vi "pressSensorLin.vi"(0 "frame":u8[](array[numeric])) -> ()   [LabVIEW 2021]
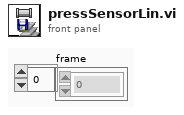
[diagram p1: front panel]
types:
  T1 = cluster{"ValvePos1":sgl, "ValvePos2":sgl, "PressureArray":sgl[], "TempArray2":sgl[], "TempArray1":sgl[], "Valve 1 Time Stamp":timestamp, "Temp 2 Array Time Stamp":timestamp[], "Temp 1 Array Time Stamp":timestamp[], "Valve 2 Time Stamp":timestamp, "Press Array Time Stamp":timestamp[]}
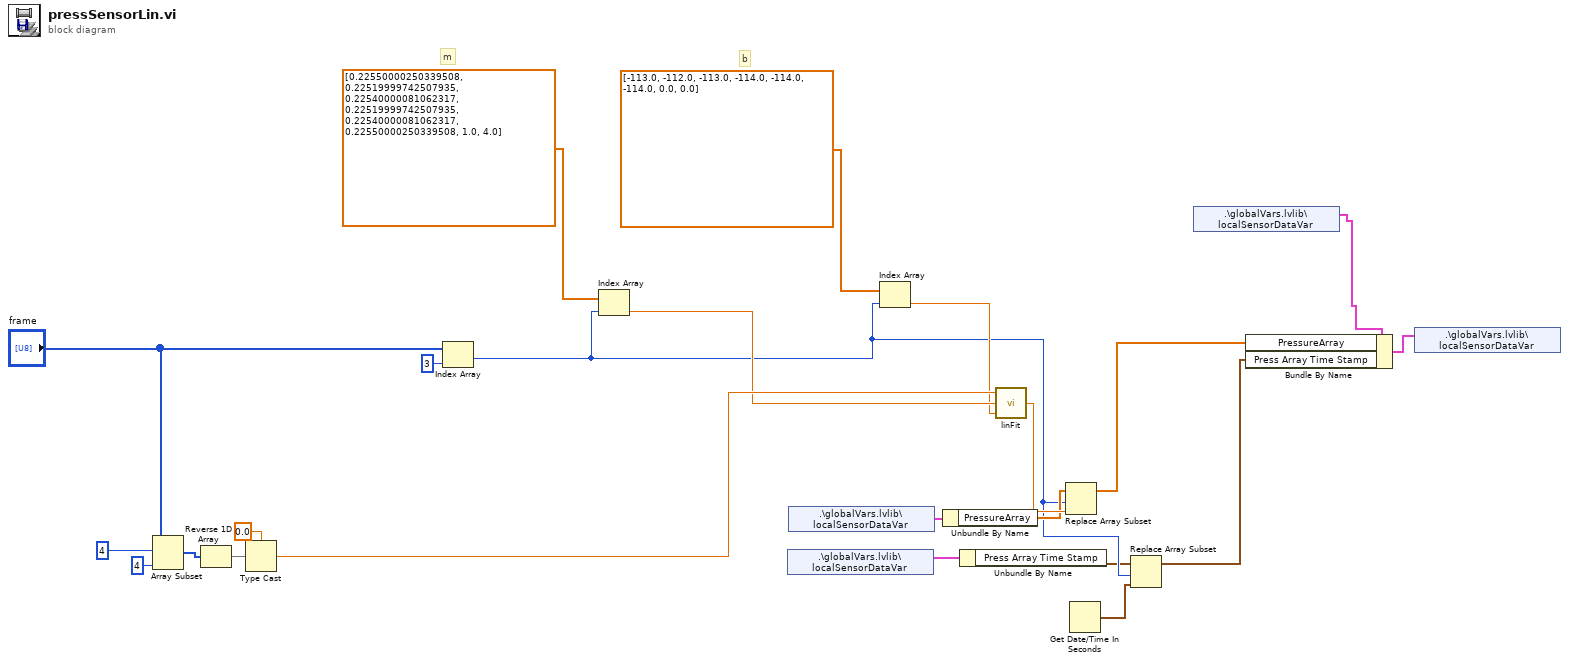
[diagram p0: block diagram]
diagram:
  # "b"
  # "m"
  n1 = Array Subset(array="frame", index=4, length=4) -> (w19:u8[])
  n2 = Reverse 1D Array(array=w19) -> (reversed array=w20:u8[])
  n3 = Type Cast(type=sgl 0.0, x=w20) -> (*(type *) &x=w14:sgl)
  n4 = Index Array(array="frame", index=3) -> (element=w5:u8)
  n5 = Index Array(array=sgl[] [0.2255, 0.2252, 0.2254, 0.2252, 0.2254, 0.2255, 1.0, 4.0], index=w5) -> (element=w13:sgl)
  n6 = shared-variable ".\\globalVars.lvlib\\localSensorDataVar"() -> (w6:T1)  [unwired: 1 in, 1 out]
  n7 = shared-variable ".\\globalVars.lvlib\\localSensorDataVar"() -> (w11:T1)  [unwired: 1 in, 1 out]
  n8 = Index Array(array=sgl[] [-113.0, -112.0, -113.0, -114.0, -114.0, -114.0, 0.0, 0.0], index=w5) -> (element=w12:sgl)
  n9 = Unbundle By Name(w11) -> ("PressureArray"=w9:sgl[])
  n10 = Unbundle By Name(w6) -> ("Press Array Time Stamp"=w3:timestamp[])
  n11 = call "linFit.vi"("b"=w12, "m"=w13, "x"=w14) -> ("xm+b"=w10:sgl)
  n12 = Replace Array Subset(array=w9, new element=w10, index=w5) -> (w8:sgl[])
  n13 = Get Date/Time In Seconds() -> (seconds since 1Jan1904=w4:timestamp)
  n14 = Replace Array Subset(array=w3, new element=w4, index=w5) -> (w2:timestamp[])
  n15 = shared-variable ".\\globalVars.lvlib\\localSensorDataVar"() -> (w1:T1)  [unwired: 1 in, 1 out]
  n16 = Bundle By Name(cluster=w1, "PressureArray"=w8, "Press Array Time Stamp"=w2) -> (w7:T1)
  n17 = shared-variable ".\\globalVars.lvlib\\localSensorDataVar"(w7) -> ()  [unwired: 1 in, 1 out]
